vi "Handix FPGA Server-80MHz.vi"() -> ()   [LabVIEW 2015]
doc: "This is the FPGA server for the sbRIO for the open-path cavity ring down."
uses:
  Rate.ctl
  <vilib>/Platform/TimedLoop/XDataNode/timing_clust.ctl
  <vilib>/Platform/TimedLoop/XDataNode/nitl_modes.ctl
  <vilib>/Platform/TimedLoop/XDataNode/wakeup.ctl
  <vilib>/rvi/FXPMathLib/FxpDiv/subVIs/nifxpmath_Div_SimConfig.ctl
  <vilib>/rvi/FXPMathLib/basic elements/FxpIntAccumulator/subVIs/nifxpmath_IntAccumulator_SimConfig.ctl
  <vilib>/rvi/Emulation/niFpgaGetClockAttributes.vi
  <vilib>/rvi/Emulation/niFpgaSctlEmulationGetInTimedLoop.vi
  <vilib>/rvi/Emulation/niFpgaEmulationReportErrorSimple.vi
  <vilib>/rvi/Emulation/niFpgaProcessEmulError.vi
  <vilib>/rvi/eio/common/nirviEmuTemplateMethod_errors.vi
  <vilib>/rvi/Emulation/niFpgaCriticalErrorInLSC.vi
  <vilib>/rvi/Analysis/common/codeGenErrors/XNode/niFpgaXNodeCodeGenErrorHandle.vi
  <vilib>/rvi/FXPMathLib/basic elements/FxpIntAccumulator/simVIs/DllFxpIntAccumulator_sub.vi
  <vilib>/rvi/FXPMathLib/FxpDiv/simVIs/DllFxpDivTemp_sub.vi
  <vilib>/rvi/interface/RandomDataEmulation/niFpgaRandomDataHandleErrors.vi
  <vilib>/eio/EIONode/EIONode.xnode
  <vilib>/rvi/Analysis/measure/mean-var-std/XNode/niFpgaMean-Var-Std.xnode
  <vilib>/Platform/TimedLoop/XDataNode/XDataNode.xnode
  <vilib>/rvi/FXPMathLib/basic elements/FxpIntAccumulator/XNode/nifxpmath_IntAccumulator.xnode
  <vilib>/rvi/FXPMathLib/FxpMul/XNode/nifxpmath_Multiplier.xnode
  <vilib>/rvi/FXPMathLib/FxpSub/XNode/nifxpmath_Sub.xnode
  <vilib>/rvi/FXPMathLib/FxpAdd/XNode/nifxpmath_Add.xnode
  <vilib>/rvi/FXPMathLib/FxpDiv/XNode/nifxpmath_Div.xnode
  <vilib>/rvi/DataTransferAndStorage/Container/XNode/niFpgaContainer.xnode
  <vilib>/rvi/interface/RandomDataEmulation/nirviRandomDataFpgaReadWriteTemplate.vi
  <vilib>/Platform/TimedLoop/XDataNode/XDNodeRunTimeDep.lvlib
  <vilib>/rvi/FXPMathLib/sim/FxpSim.dll
panel:
  in  "u_offset":fxp<+/-,32,16>=-2.5
  in  "theated_offset":fxp<+/-,32,16>=-250.0
  in  "theated_slope":fxp<+/-,32,16>=200.0
  in  "p_offset":fxp<+/-,32,16>=-3.0
  in  "p_slope":fxp<+/-,32,16>=2.0
  in  "u_slope":fxp<+/-,32,16>=2.5099945068359375
  out "pressure (mb)":fxp<+/-,32,12>
  in  "Heater Input":fxp<+/-,20,5>
  out "uplenum":fxp<+/-,24,12>
  out "Theatedline":fxp<+/-,24,12>
  out "Thermistor Data":T1
  in  "Primary Vol Fan":fxp<+/-,20,5>
  in  "KNF Pump":fxp<+/-,20,5>
  out "ServoLoop":bool
  in  "Low":u32 caption="Count(uSec)"
  in  "High":u32 caption="Count(uSec)"
  out "Vaisala":T2
  out "CollectData":bool
  in  "InvertLaser?":bool
  in  "LaserOff (us)":u32
  in  "Fans":T3
  in  "Reverse?":bool
  out "EncodeLoop":bool
  out "LaserLoop":bool
  out "HKLoop":bool
  out "DataLoop":bool
  out "Delay Ticks":u32
  in  "Delay (us)":u16
  out "RequestLaser":bool
  out "Sample Ticks":u32
  in  "Pause Digitizer":bool
  in  "Sample Time (us)":u16
  in  "Rate":T4=3 items=["1 MHz"=20, "2 MHz"=10, "2.5 MHz"=8, "5 MHz"=4, "10 MHz"=2, "20MHz"=1]
  out "LaserOFF?":bool
  in  "Cylce (ticks)":u32=40000
  out "NumElements":u32
  in  "Stop":bool
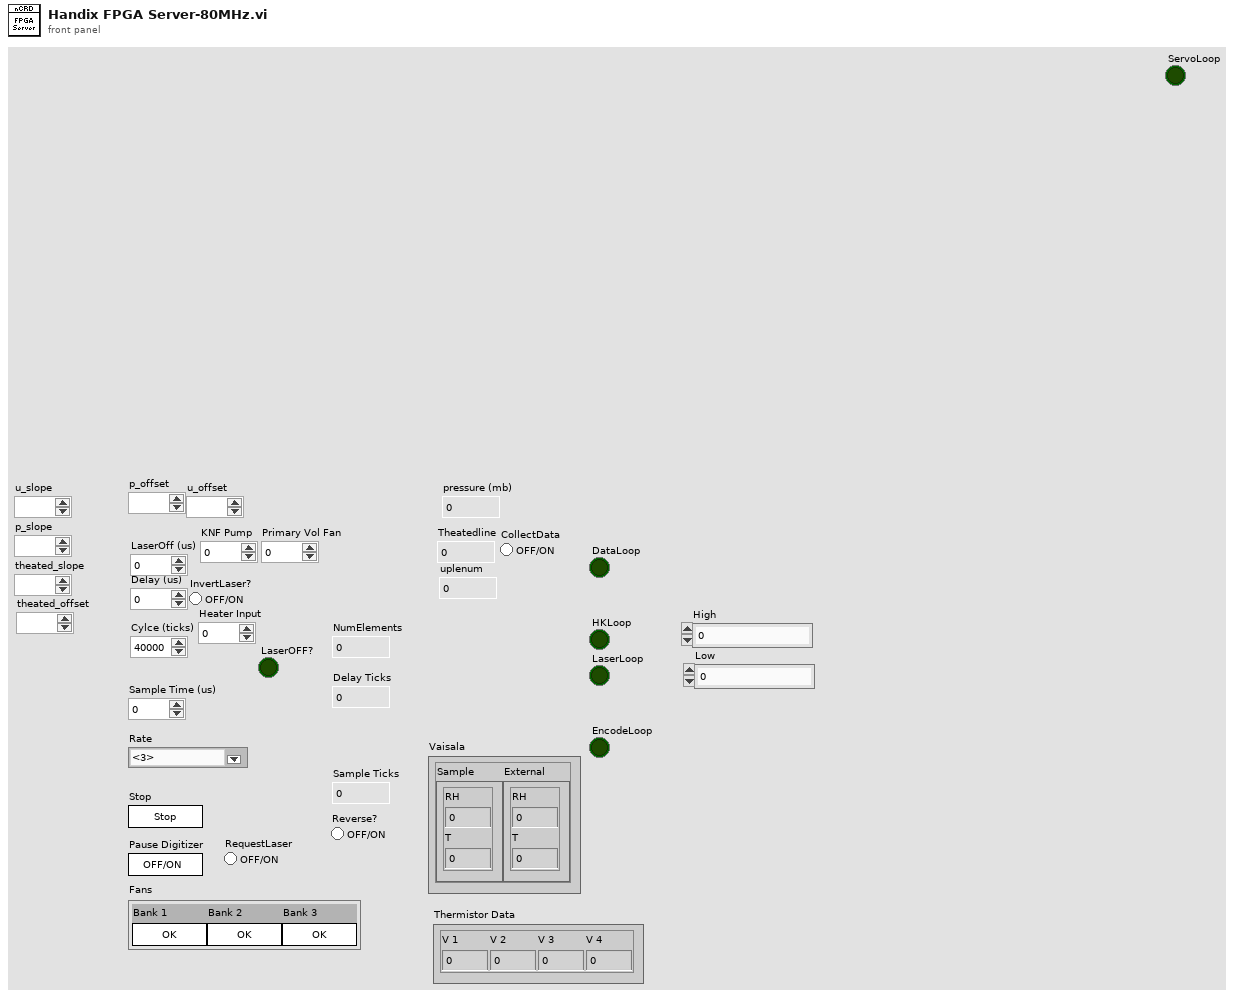
[diagram p1: front panel]
types:
  T1 = cluster{"V 1":fxp<+/-,24,5>, "V 2":fxp<+/-,24,5>, "V 3":fxp<+/-,24,5>, "V 4":fxp<+/-,24,5>}
  T2 = cluster{"Sample":cluster{"RH":fxp<+,16,8>, "T":fxp<+/-,16,8>}, "External":cluster{"RH":fxp<+,16,8>, "T":fxp<+/-,16,8>}}
  T3 = cluster{"Bank 1":bool, "Bank 2":bool, "Bank 3":bool}
  T4 = typedef "Rate.ctl" = u8
  T5 = typedef "XDNodeRunTimeDep.lvlib/timing_clust.ctl" = cluster{"Expected End [f-1]":u64, "Actual End [f-1]":u64, "Finished Late? [f-1]":bool, "Expected End [i-1]":u64, "Actual End [i-1]":u64, "Finished Late? [i-1]":bool, "Expected Start [i]":u64, "Actual Start [i]":u64, "Expected Start [f]":u64, "Actual Start [f]":u64, "Source Name":string, "Structure Name":string, "Period":i64, "Deadline":i64, "Offset":i64, "Start":i64, "Priority":i32, "Timeout":i32, "Mode":T6, "Wakeup Reason":T7, "Error":errorcluster, "Source Type":string, "Secondary Source Type":string, "Global End Time":u64, "Global Start Time":u64, "Frame Duration":u64, "Iteration Duration":u64, "Assigned CPU":i32, "I/O Scan Engine Mode":u32}
  T6 = typedef "XDNodeRunTimeDep.lvlib/nitl_modes.ctl" = enum32{"No Change", "Process missed periods, maintain original phase", "Discard missed periods, maintain original phase", "Process missed periods, ignore original phase", "Discard missed periods, ignore original phase"}
  T7 = typedef "XDNodeRunTimeDep.lvlib/wakeup.ctl" = enum32{"Normal", "Aborted", "Asynchronous wakeup", "Timing source error", "Timed loop error", "Timeout"}
  T8 = cluster{"mean":fxp<+/-,24,5>, "mean":fxp<+/-,24,5>, "mean":fxp<+/-,24,5>, "mean":fxp<+/-,24,5>}
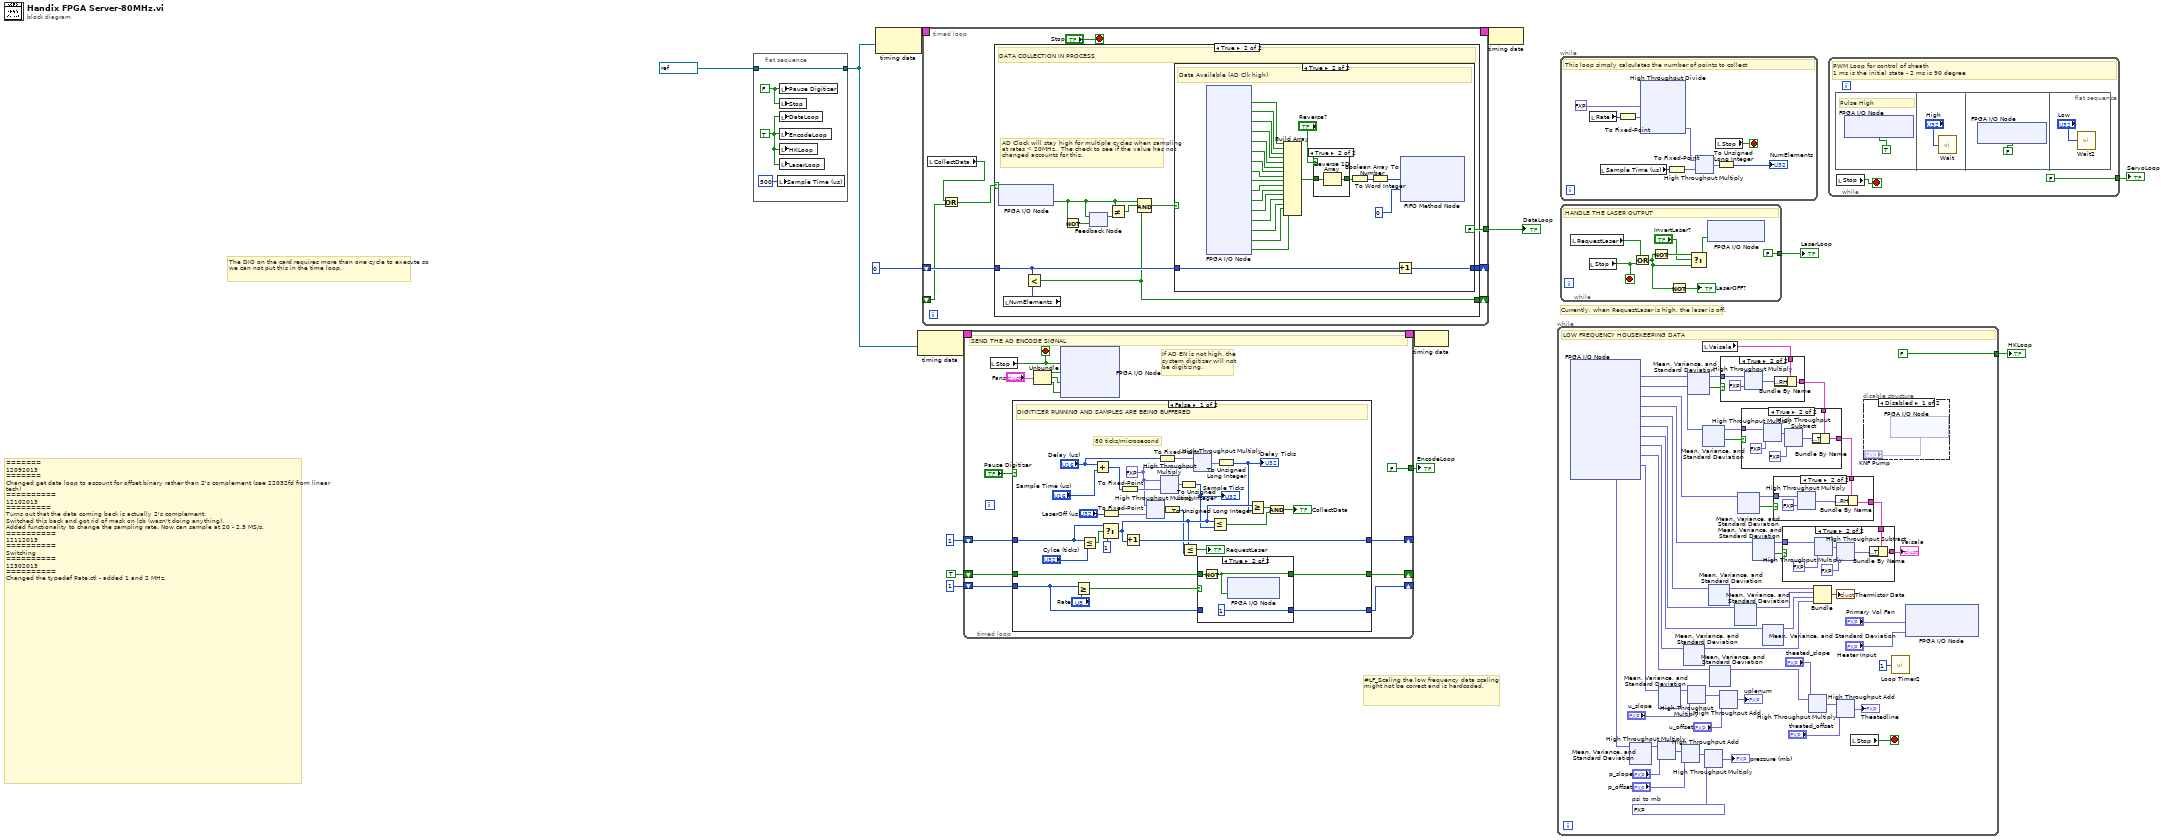
[diagram p0: block diagram]
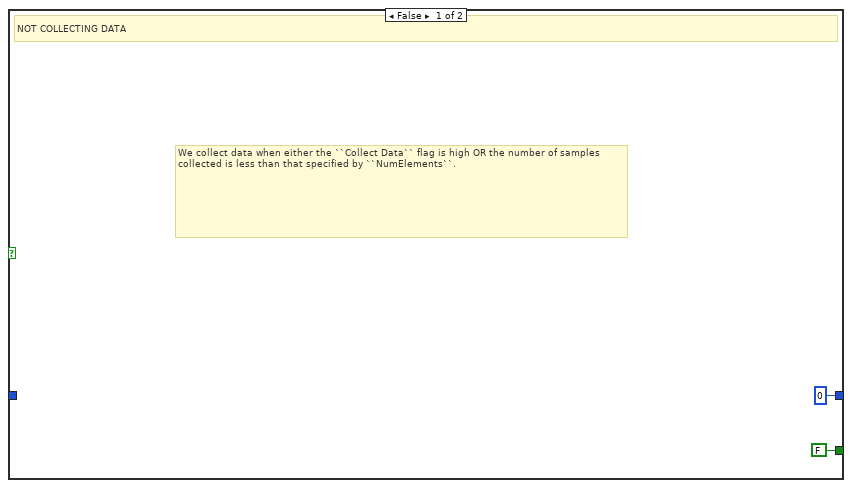
[diagram p2: hidden frame]
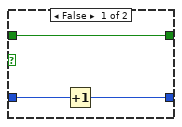
[diagram p10: hidden frame]
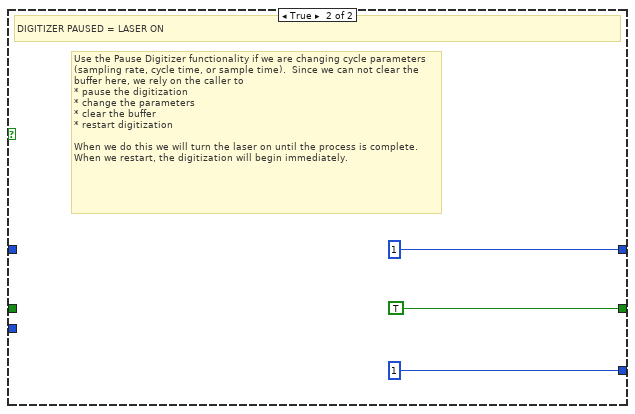
[diagram p11: hidden frame]
diagram:
  # "Currently, when RequestLaser is high, the laser is off."
  # "#LF_Scaling the low frequency data scaling might not be correct and is hardcoded."
  # "The DIO on the card requires more than one cycle to execute so we can not put this in the time loop."
  # "=======\n12092013 \n=======\nChanged get data loop to account for offset binary rather than 2's complement (see 22032fd from linear tech)\n==========\n12102013\n=========\nTurns out that the data coming back is actually 2's complement. \nSwitched this back and got rid of mask on lsb (wasn't doing anything).\nAdded functionality to change the sampling rate. Now can sample at 20 - 2.5 MS/s.\n==========\n12112013\n==========\nSwitching\n==========\n12302013\n==========\nChanged the typedef Rate.ctl - added 1 and 2 MHz."
  n1 = flat-sequence {
    tunnel: refnum<k21> "80MHz" ("Source Name") -> [w19]
    tunnel: [w19] -> w2
    frame #0 {
      w17 = TRUE
      w18 = FALSE ("Pause Digitizer")
      n2 = local write "Sample Time (us)"(u16 500 ("Sample Time (us)")) -> ()
      n3 = local write "Pause Digitizer"(w18) -> ()
      n4 = local write "Stop"(w18) -> ()
      n5 = local write "DataLoop"(w17) -> ()
      n6 = local write "EncodeLoop"(w17) -> ()
      n7 = local write "HKLoop"(w17) -> ()
      n8 = local write "LaserLoop"(w17) -> ()
    }
  }
  n9 = node-c288(w2) -> (w6:T5)
  n10 = node-c288(w2) -> (w15:T5)
  n11 = timed-loop {
    timing: w6 -> [_]
    timing-out: [_] -> w5
    shift-right: [w27] -> _
    shift-left: u32 0 -> [w26]
    tunnel: [FALSE] -> w3
    shift-right: [w21] -> _
    shift-left: _ -> [w20]
    stop <- "Stop" stop-if-true
    n12 = local read "CollectData"() -> (w23:bool)
    n13 = Or(x=w23, y=w20) -> (x .or. y?=w22:bool)
    n14 = case shown="True" w22 {
      tunnel: [u32 0 w38] -> w27
      tunnel: w26 -> [_ w37]
      tunnel: [FALSE w30] -> w21
      frame False {
        # "We collect data when either the ``Collect Data`` flag is high OR the number of samples collected is less than that specified by ``NumElements``."
        # "NOT COLLECTING DATA"
      }
      frame True {
        # "AD Clock will stay high for multiple cycles when sampling at rates < 20MHz.  The check to see if the value has not changed accounts for this."
        # "DATA COLLECTION IN PROCESS"
        n15 = xnode "FPGA I/O Node"() -> ("AD CLK +"=w32:bool)  [unwired: 1 in, 1 out]
        n16 = local read "NumElements"() -> (w36:u32)
        n17 = Less?(x=w37, y=w36) -> (x < y?=w30:bool)
        n18 = Not(x=w32) -> (.not. x?=w34:bool)
        n19 = feedback #1(w34) -> (w35:bool)
        n20 = feedback-in #1(w32) -> ()
        n21 = Not Equal?(x=w32, y=w35) -> (x != y?=w33:bool)
        n22 = Compound Arithmetic op=AND(w32, w33, w30) -> (w31:bool)
        n23 = case shown="True" w31 {
          tunnel: w37 -> [w39 w43]
          tunnel: [w39 w44] -> w38
          frame False {
            # "Waiting (Clk previously high or currently low)"
          }
          frame True {
            # "Data Available (AD Clk high)"
            n24 = xnode "FPGA I/O Node"() -> ("AD0"=w45:bool, "AD1"=w46:bool, "AD2"=w47:bool, "AD3"=w48:bool, "AD4"=w49:bool, "AD5"=w50:bool, "AD6"=w51:bool, "AD7"=w52:bool, "AD8"=w53:bool, "AD9"=w54:bool, "AD10"=w55:bool, "AD11"=w56:bool, "AD12"=w57:bool, "AD13"=w58:bool, "AD14"=w59:bool, "AD15"=w60:bool)  [unwired: 16 in, 16 out]
            n25 = Build Array(w45, w46, w47, w48, w49, w50, w51, w52, w53, w54, w55, w56, w57, w58, w59, w60) -> (w62:bool[])
            n26 = case shown="True" "Reverse?" {
              tunnel: w62 -> [w64 w66]
              tunnel: [w64 w65] -> w63
              frame False {
              }
              frame True {
                n27 = Reverse 1D Array(array=w66) -> (reversed array=w65:bool[])
              }
            }
            n28 = Boolean Array To Number(Boolean array=w63) -> (number=w61:u16)
            n29 = To Word Integer(number=w61) -> (16bit integer=w41:i16)
            n30 = Increment(x=w43) -> (x+1=w44:u32)
            n31 = xnode ("FIFO Method Node")("Element"=w41, "Timeout"=0) -> ()  [unwired: 1 in, 2 out]
          }
        }
      }
    }
  }
  "DataLoop" <- w3
  n32 = timed-loop {
    shift-right: [w77] -> _
    shift-left: TRUE -> [w78]
    timing: w15 -> [_]
    timing-out: [_] -> w14
    shift-right: [w79] -> _
    shift-left: u32 1 -> [w80]
    shift-right: [w76] -> _
    shift-left: u8 1 -> [w75]
    tunnel: [FALSE] -> w7
    stop <- w81 stop-if-true
    # "If AD EN is not high, the system digitizer will not be digitizing."
    # "SEND THE AD ENCODE SIGNAL"
    n33 = local read "Stop"() -> (w81:bool)
    n34 = case shown="False" "Pause Digitizer" {
      tunnel: w80 -> [w94 _]
      tunnel: [w109 u32 1] -> w79
      tunnel: w78 -> [w106 _]
      tunnel: [w105 TRUE ("Element")] -> w77
      tunnel: [w104 u8 1] -> w76
      tunnel: w75 -> [w103 _]
      frame False {
        w90 = fxp<+,8,8> 80.0 ("Sample Time (us) 2")
        # "80 ticks/microsecond"
        # "DIGITIZER RUNNING AND SAMPLES ARE BEING BUFFERED"
        n35 = Greater Or Equal?(x=w103, y="Rate") -> (x >= y?=w107:bool)
        n36 = Less Or Equal?(x=w94, y="Cylce (ticks)") -> (x <= y?=w111:bool)
        n37 = Add(x="Delay (us)", y="Sample Time (us)") -> (x+y=w100:u16)
        n38 = Select(t=w94, s=w111, f=u32 1) -> (s? t:f=w92:u32)
        n39 = To Fixed-Point(number="LaserOff (us)") -> (fixed-point=w88:fxp<+,32,32>)  [unwired: 1 in]
        n40 = To Fixed-Point(number=w100) -> (fixed-point=w101:fxp<+,16,16>)  [unwired: 1 in]
        n41 = Increment(x=w92) -> (x+1=w109:u32)
        n42 = xnode ("High Throughput Multiply")("x"=w90, "y"=w88) -> ("x*y"=w87:fxp<+,32,32>)
        n43 = To Fixed-Point(number="Delay (us)") -> (fixed-point=w97:fxp<+,16,16>)  [unwired: 1 in]
        n44 = xnode ("High Throughput Multiply")("x"=w90, "y"=w101) -> ("x*y"=w102:fxp<+,32,32>)
        n45 = To Unsigned Long Integer(number=w87) -> (unsigned 32bit integer=w86:u32)
        n46 = To Unsigned Long Integer(number=w102) -> (unsigned 32bit integer=w82:u32)
        "Sample Ticks" <- w82
        n47 = Less Or Equal?(x=w92, y=w86) -> (x <= y?=→"RequestLaser":bool)
        n48 = xnode ("High Throughput Multiply")("x"=w97, "y"=w90) -> ("x*y"=w96:fxp<+,32,32>)
        n49 = case shown="True" w107 {
          tunnel: w106 -> [w114 w117]
          tunnel: [w114 w116] -> w105
          tunnel: [w112 u8 1] -> w104
          tunnel: w103 -> [w113 _]
          frame False {
            n50 = Increment(x=w113) -> (x+1=w112:u8)
          }
          frame True {
            n51 = Not(x=w117) -> (.not. x?=w116:bool)
            n52 = xnode "FPGA I/O Node"("ENCODE"=w116) -> ()  [unwired: 1 in, 1 out]
          }
        }
        n53 = Less Or Equal?(x=w92, y=w82) -> (x <= y?=w99:bool)
        n54 = To Unsigned Long Integer(number=w96) -> (unsigned 32bit integer=w83:u32)
        "Delay Ticks" <- w83
        n55 = Greater Or Equal?(x=w92, y=w83) -> (x >= y?=w95:bool)
        n56 = And(x=w95, y=w99) -> (x .and. y?=→"CollectData":bool)
      }
      frame True {
        # "Use the Pause Digitizer functionality if we are changing cycle parameters (sampling rate, cycle time, or sample time).  Since we can not clear the buffer here, we rely on the caller to \n* pause the digitization\n* change the parameters\n* clear the buffer\n* restart digitization\n\nWhen we do this we will turn the laser on until the process is complete. When we restart, the digitization will begin immediately."
        # "DIGITIZER PAUSED = LASER ON"
      }
    }
    n57 = Unbundle("Fans") -> ("Bank 1"=w71:bool, "Bank 2"=w70:bool, "Bank 3"=w69:bool)
    n58 = xnode "FPGA I/O Node"("AD EN"=w81, "Fan Bank 4"=w71, "Fan Bank 2"=w70, "Fan Bank 3"=w69) -> ()  [unwired: 4 in, 4 out]
  }
  "EncodeLoop" <- w7
  n59 = node-c288(w14) -> ()
  n60 = node-c288(w5) -> ()
  n61 = while {
    tunnel: [FALSE] -> w9
    stop <- w166 stop-if-true
    w136 = fxp<+,32,8> 68.94757282733917  # psi to mb
    # "LOW FREQUENCY HOUSEKEEPING DATA"
    n62 = xnode "FPGA I/O Node"() -> ("External RH"=w172:fxp<+/-,24,5>, "External Temp"=w171:fxp<+/-,24,5>, "Sample RH"=w164:fxp<+/-,24,5>, "Sample Temp"=w163:fxp<+/-,24,5>, "Temperature 1"=w152:fxp<+/-,24,5>, "Temperature 2"=w151:fxp<+/-,24,5>, "Temperature 3"=w150:fxp<+/-,24,5>, "Temperature 4"=w149:fxp<+/-,24,5>, "Theatedline"=w142:fxp<+/-,24,5>, "uplenum"=w143:fxp<+/-,24,5>, "Pressure"=w138:fxp<+/-,24,5>)  [unwired: 11 in, 11 out]
    n63 = xnode "Mean, Variance, and Standard Deviation"("input data"=w138) -> ("mean"=w134:fxp<+/-,24,5>)  [unwired: 1 in, 1 out]
    n64 = xnode "High Throughput Multiply"("x"=w134, "y"="p_slope") -> ("x*y"=w132:fxp<+/-,56,21>)
    n65 = xnode "Mean, Variance, and Standard Deviation"("input data"=w143) -> ("mean"=w139:fxp<+/-,24,5>)  [unwired: 1 in, 1 out]
    n66 = xnode "High Throughput Add"("x"=w132, "y"="p_offset") -> ("x+y"=w137:fxp<+/-,57,22>)
    n67 = xnode "Mean, Variance, and Standard Deviation"("input data"=w149) -> ("mean"=w145:fxp<+/-,24,5>)  [unwired: 1 in, 1 out]
    n68 = xnode "High Throughput Multiply"("x"=w139, "y"="u_slope") -> ("x*y"=w125:fxp<+/-,56,21>)
    n69 = xnode "Mean, Variance, and Standard Deviation"("input data"=w172) -> ("mean"=w170:fxp<+/-,24,5>, "output valid"=w169:bool)  [unwired: 1 in]
    n70 = local read "Vaisala"() -> (w158:T2)
    n71 = xnode "Mean, Variance, and Standard Deviation"("input data"=w171) -> ("mean"=w167:fxp<+/-,24,5>, "output valid"=w168:bool)  [unwired: 1 in]
    n72 = xnode "High Throughput Multiply"("x"=w137, "y"=w136) -> ("x*y"=→"pressure (mb)":fxp<+/-,32,12>)
    n73 = xnode "Mean, Variance, and Standard Deviation"("input data"=w152) -> ("mean"=w148:fxp<+/-,24,5>)  [unwired: 1 in, 1 out]
    n74 = xnode "Mean, Variance, and Standard Deviation"("input data"=w142) -> ("mean"=w129:fxp<+/-,24,5>)  [unwired: 1 in, 1 out]
    n75 = xnode "High Throughput Add"("x"=w125, "y"="u_offset") -> ("x+y"=→"uplenum":fxp<+/-,24,12>)
    n76 = case shown="True" w169 {
      tunnel: w170 -> [_ w885]
      tunnel: w158 -> [w881 w884]
      tunnel: [w881 w883] -> w157
      frame False {
      }
      frame True {
        n77 = xnode ("High Throughput Multiply")("x"=w885, "y"=fxp<+,8,8> 20.0) -> ("x*y"=w882:fxp<+,16,8>)
        n78 = Bundle By Name(cluster=w884, "External.RH"=w882) -> (w883:T2)
      }
    }
    n79 = xnode "Mean, Variance, and Standard Deviation"("input data"=w151) -> ("mean"=w147:fxp<+/-,24,5>)  [unwired: 1 in, 1 out]
    n80 = xnode "Mean, Variance, and Standard Deviation"("input data"=w164) -> ("mean"=w162:fxp<+/-,24,5>, "output valid"=w161:bool)  [unwired: 1 in]
    n81 = case shown="True" w168 {
      tunnel: w167 -> [_ w877]
      tunnel: w157 -> [w873 w876]
      tunnel: [w873 w875] -> w156
      frame False {
      }
      frame True {
        n82 = xnode ("High Throughput Multiply")("x"=w877, "y"=fxp<+,8,8> 20.0) -> ("x*y"=w879:fxp<+/-,32,13>)
        n83 = xnode "High Throughput Subtract"("x"=w879, "y"=fxp<+/-,8,8> 40.0) -> ("x-y"=w874:fxp<+/-,16,8>)
        n84 = Bundle By Name(cluster=w876, "External.T"=w874) -> (w875:T2)
      }
    }
    n85 = xnode "Mean, Variance, and Standard Deviation"("input data"=w163) -> ("mean"=w160:fxp<+/-,24,5>, "output valid"=w159:bool)  [unwired: 1 in]
    n86 = xnode "Mean, Variance, and Standard Deviation"("input data"=w150) -> ("mean"=w146:fxp<+/-,24,5>)  [unwired: 1 in, 1 out]
    n87 = case shown="True" w161 {
      tunnel: w162 -> [_ w719]
      tunnel: w156 -> [w715 w718]
      tunnel: [w715 w717] -> w155
      frame False {
      }
      frame True {
        n88 = xnode ("High Throughput Multiply")("x"=w719, "y"=fxp<+,8,8> 20.0) -> ("x*y"=w716:fxp<+,16,8>)
        n89 = Bundle By Name(cluster=w718, "Sample.RH"=w716) -> (w717:T2)
      }
    }
    n90 = case shown="True" w159 {
      tunnel: w160 -> [_ w711]
      tunnel: w155 -> [w707 w710]
      tunnel: [w707 w709] -> w154
      frame False {
      }
      frame True {
        n91 = xnode ("High Throughput Multiply")("x"=w711, "y"=fxp<+,8,8> 20.0) -> ("x*y"=w713:fxp<+/-,32,13>)
        n92 = xnode "High Throughput Subtract"("x"=w713, "y"=fxp<+/-,8,8> 40.0) -> ("x-y"=w708:fxp<+/-,16,8>)
        n93 = Bundle By Name(cluster=w710, "Sample.T"=w708) -> (w709:T2)
      }
    }
    "Vaisala" <- w154
    n94 = xnode "High Throughput Multiply"("x"=w129, "y"="theated_slope") -> ("x*y"=w130:fxp<+/-,56,21>)
    n95 = Bundle("mean"=w148, "mean"=w147, "mean"=w146, "mean"=w145) -> (→"Thermistor Data":T8)  [unwired: 1 in]
    n96 = xnode "High Throughput Add"("x"=w130, "y"="theated_offset") -> ("x+y"=→"Theatedline":fxp<+/-,24,12>)
    n97 = local read "Stop"() -> (w166:bool)
    n98 = disable-structure shown="Disabled" {
      frame Disabled {
        n99 = xnode "FPGA I/O Node"("KNF Pump"="KNF Pump") -> ()  [unwired: 1 in, 1 out]
      }
      frame Enabled {
      }
    }
    n100 = call "Loop Timer2"("Count(mSec)"=u32 1 ("Count(Ticks)")) -> ()  [unwired: 1 out]
    n101 = xnode "FPGA I/O Node"("Primary Vol Fan"="Primary Vol Fan", "Heater"="Heater Input") -> ()  [unwired: 2 in, 2 out]
  }
  "HKLoop" <- w9
  n102 = while {
    stop <- w1047 stop-if-true
    # "This loop simply calculates the number of points to collect"
    n103 = local read "Rate"() -> (w1043:T4)
    n104 = local read "Sample Time (us)"() -> (w1046:u16)
    n105 = To Fixed-Point(number=w1043) -> (fixed-point=w1042:fxp<+,8,8>)  [unwired: 1 in]
    n106 = xnode "High Throughput Divide"("x"=fxp<+,8,8> 40.0 ("Sample Time (us) 2"), "y"=w1042) -> ("x/y"=w1041:fxp<+,16,8>)
    n107 = To Fixed-Point(number=w1046) -> (fixed-point=w1045:fxp<+,16,16>)  [unwired: 1 in]
    n108 = xnode ("High Throughput Multiply")("x"=w1041, "y"=w1045) -> ("x*y"=w1040:fxp<+,32,32>)
    n109 = local read "Stop"() -> (w1047:bool)
    n110 = To Unsigned Long Integer(number=w1040) -> (unsigned 32bit integer=→"NumElements":u32)
  }
  n111 = while {
    tunnel: [FALSE] -> w8
    stop <- w1081 stop-if-true
    # "HANDLE THE LASER OUTPUT"
    n112 = local read "RequestLaser"() -> (w1082:bool)
    n113 = local read "Stop"() -> (w1081:bool)
    n114 = Or(x=w1082, y=w1081) -> (x .or. y?=w1076:bool)
    n115 = Not(x=w1076) -> (.not. x?=w1078:bool)
    n116 = Not(x=w1076) -> (.not. x?=→"LaserOFF?":bool)
    n117 = Select(t=w1078, s="InvertLaser?", f=w1076) -> (s? t:f=w1077:bool)
    n118 = xnode "FPGA I/O Node"("Laser Mod"=w1077) -> ()  [unwired: 1 in, 1 out]
  }
  "LaserLoop" <- w8
  n119 = while {
    tunnel: [FALSE] -> w1
    stop <- w1083 stop-if-true
    # "PWM Loop for control of sheath\n1 ms is the initial state - 2 ms is 90 degree"
    n120 = flat-sequence {
      frame #0 {
        # "Pulse High"
        n121 = xnode "FPGA I/O Node"("Motor Control"=TRUE ("Mod4/DIO0")) -> ()  [unwired: 1 in, 1 out]
      }
      frame #1 {
        n122 = call "Wait"("Count(uSec)"="High") -> ()  [unwired: 1 out]
      }
      frame #2 {
        n123 = xnode "FPGA I/O Node"("Motor Control"=FALSE ("Mod4/DIO0")) -> ()  [unwired: 1 in, 1 out]
      }
      frame #3 {
        n124 = call "Wait2"("Count(Ticks)"="Low") -> ()  [unwired: 1 out]
      }
    }
    n125 = local read "Stop"() -> (w1083:bool)
  }
  "ServoLoop" <- w1
